vi "Top.vi"(0 "OPC UA client refnum out":T4, 9 "stop":bool, 11 "error IO":errorcluster) -> (3 "Az":T5, 4 "Alt":T6, 6 "HSB":T7, 8 "Fork Panel":T8, 10 "UPS":T10, 15 "Alarm Error":T11)   [LabVIEW 2019]
uses:
  subVIs/Alarm-Ctrl.ctl
  subVIs/UPS-Ctrl.ctl
  <vilib>/OPCUA/controls/NodeId.ctl
  subVIs/Fork Panel-Ctrl.ctl
  subVIs/HSB-Ctrl.ctl
  subVIs/Alt-Ctrl.ctl
  subVIs/Az-Ctrl.ctl
  <vilib>/OPCUA/controls/OPC UA Client Refnum.ctl
  subVIs/Ack-Ctrl.ctl
  <vilib>/OPCUA/controls/Write Variant Request.ctl
  <vilib>/OPCUA/controls/Write Status.ctl
  <vilib>/OPCUA/client/Multiple Write Variant.vi
  <vilib>/OPCUA/NI OPC UA Client.lvlib
panel:
  in  "Alarm_Ack":T1
  in  "UPS_Ack":T2
  in  "FP_Ack":T3
  in  "HSB_Ack":T3
  in  "Alt_Ack":T3
  in  "Az_Ack":T3
  out "node RU":T9[](array[typedef])
  out "node RU 2":T9[](array[typedef])
  out "node RU 3":string[](array[string])
  # "Alarm Error"
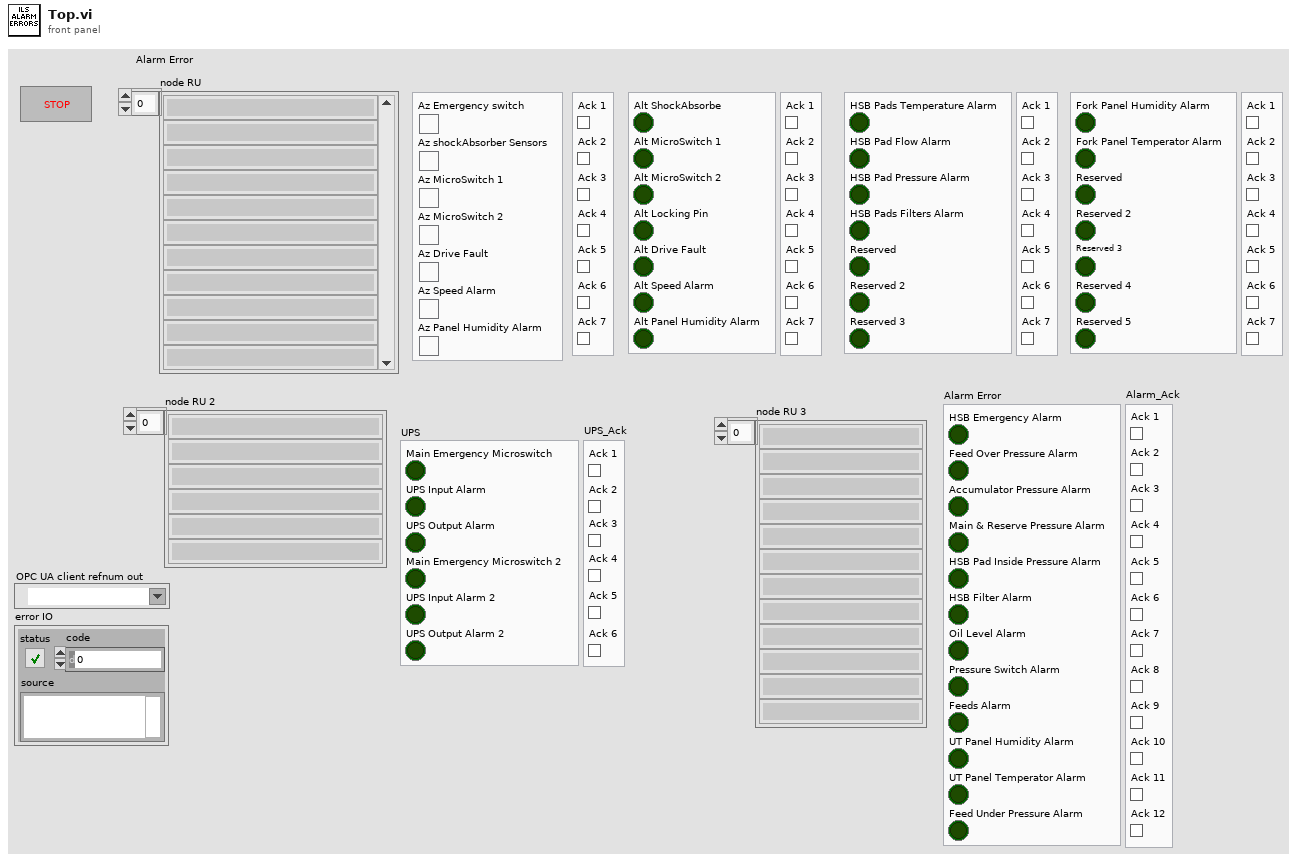
[diagram p1: front panel]
types:
  T1 = cluster{"Ack 1":bool, "Ack 2":bool, "Ack 3":bool, "Ack 4":bool, "Ack 5":bool, "Ack 6":bool, "Ack 7":bool, "Ack 8":bool, "Ack 9":bool, "Ack 10":bool, "Ack 11":bool, "Ack 12":bool}
  T2 = cluster{"Ack 1":bool, "Ack 2":bool, "Ack 3":bool, "Ack 4":bool, "Ack 5":bool, "Ack 6":bool}
  T3 = typedef "Ack-Ctrl.ctl" = cluster{"Ack 1":bool, "Ack 2":bool, "Ack 3":bool, "Ack 4":bool, "Ack 5":bool, "Ack 6":bool, "Ack 7":bool}
  T4 = typedef "OPC UA Client Refnum.ctl" = refnum<k21>
  T5 = typedef "Az-Ctrl.ctl" = cluster{"Az Emergency switch":bool, "Az shockAbsorber Sensors":bool, "Az MicroSwitch 1":bool, "Az MicroSwitch 2":bool, "Az Drive Fault":bool, "Az Speed Alarm":bool, "Az Panel Humidity Alarm":bool}
  T6 = typedef "Alt-Ctrl.ctl" = cluster{"Alt ShockAbsorbe":bool, "Alt MicroSwitch 1":bool, "Alt MicroSwitch 2":bool, "Alt Locking Pin":bool, "Alt Drive Fault":bool, "Alt Speed Alarm":bool, "Alt Panel Humidity Alarm":bool}
  T7 = typedef "HSB-Ctrl.ctl" = cluster{"HSB Pads Temperature Alarm":bool, "HSB Pad Flow Alarm":bool, "HSB Pad Pressure Alarm":bool, "HSB Pads Filters Alarm":bool, "Reserved":bool, "Reserved 2":bool, "Reserved 3":bool}
  T8 = typedef "Fork Panel-Ctrl.ctl" = cluster{"Fork Panel Humidity Alarm":bool, "Fork Panel Temperator Alarm":bool, "Reserved":bool, "Reserved 2":bool, "Reserved 3":bool, "Reserved 4":bool, "Reserved 5":bool}
  T9 = typedef "NodeId.ctl" = string
  T10 = typedef "UPS-Ctrl.ctl" = cluster{"Main Emergency Microswitch":bool, "UPS Input Alarm":bool, "UPS Output Alarm":bool, "Main Emergency Microswitch 2":bool, "UPS Input Alarm 2":bool, "UPS Output Alarm 2":bool}
  T11 = typedef "Alarm-Ctrl.ctl" = cluster{"HSB Emergency Alarm":bool, "Feed Over Pressure Alarm":bool, "Accumulator Pressure Alarm":bool, "Main & Reserve Pressure Alarm":bool, "HSB Pad Inside Pressure Alarm":bool, "HSB Filter Alarm":bool, "Oil Level Alarm":bool, "Pressure Switch Alarm":bool, "Feeds Alarm":bool, "UT Panel Humidity Alarm":bool, "UT Panel Temperator Alarm":bool, "Feed Under Pressure Alarm":bool}
  T12 = typedef "Write Variant Request.ctl" = cluster{"node ID":T9, "value":variant, "timestamp (current time)":timestamp, "node status":T13}
  T13 = typedef "Write Status.ctl" = u32
  T14 = typedef "Subscription ID.ctl" = u32
  T15 = typedef "Subscription Data Change.ctl" = cluster{"node ID":T9, " value":variant, "timestamp":timestamp, "data type":T16, "status code":T17}
  T16 = typedef "Data Type.ctl" = u16
  T17 = typedef "OPC UA StatusCode.ctl" = u32
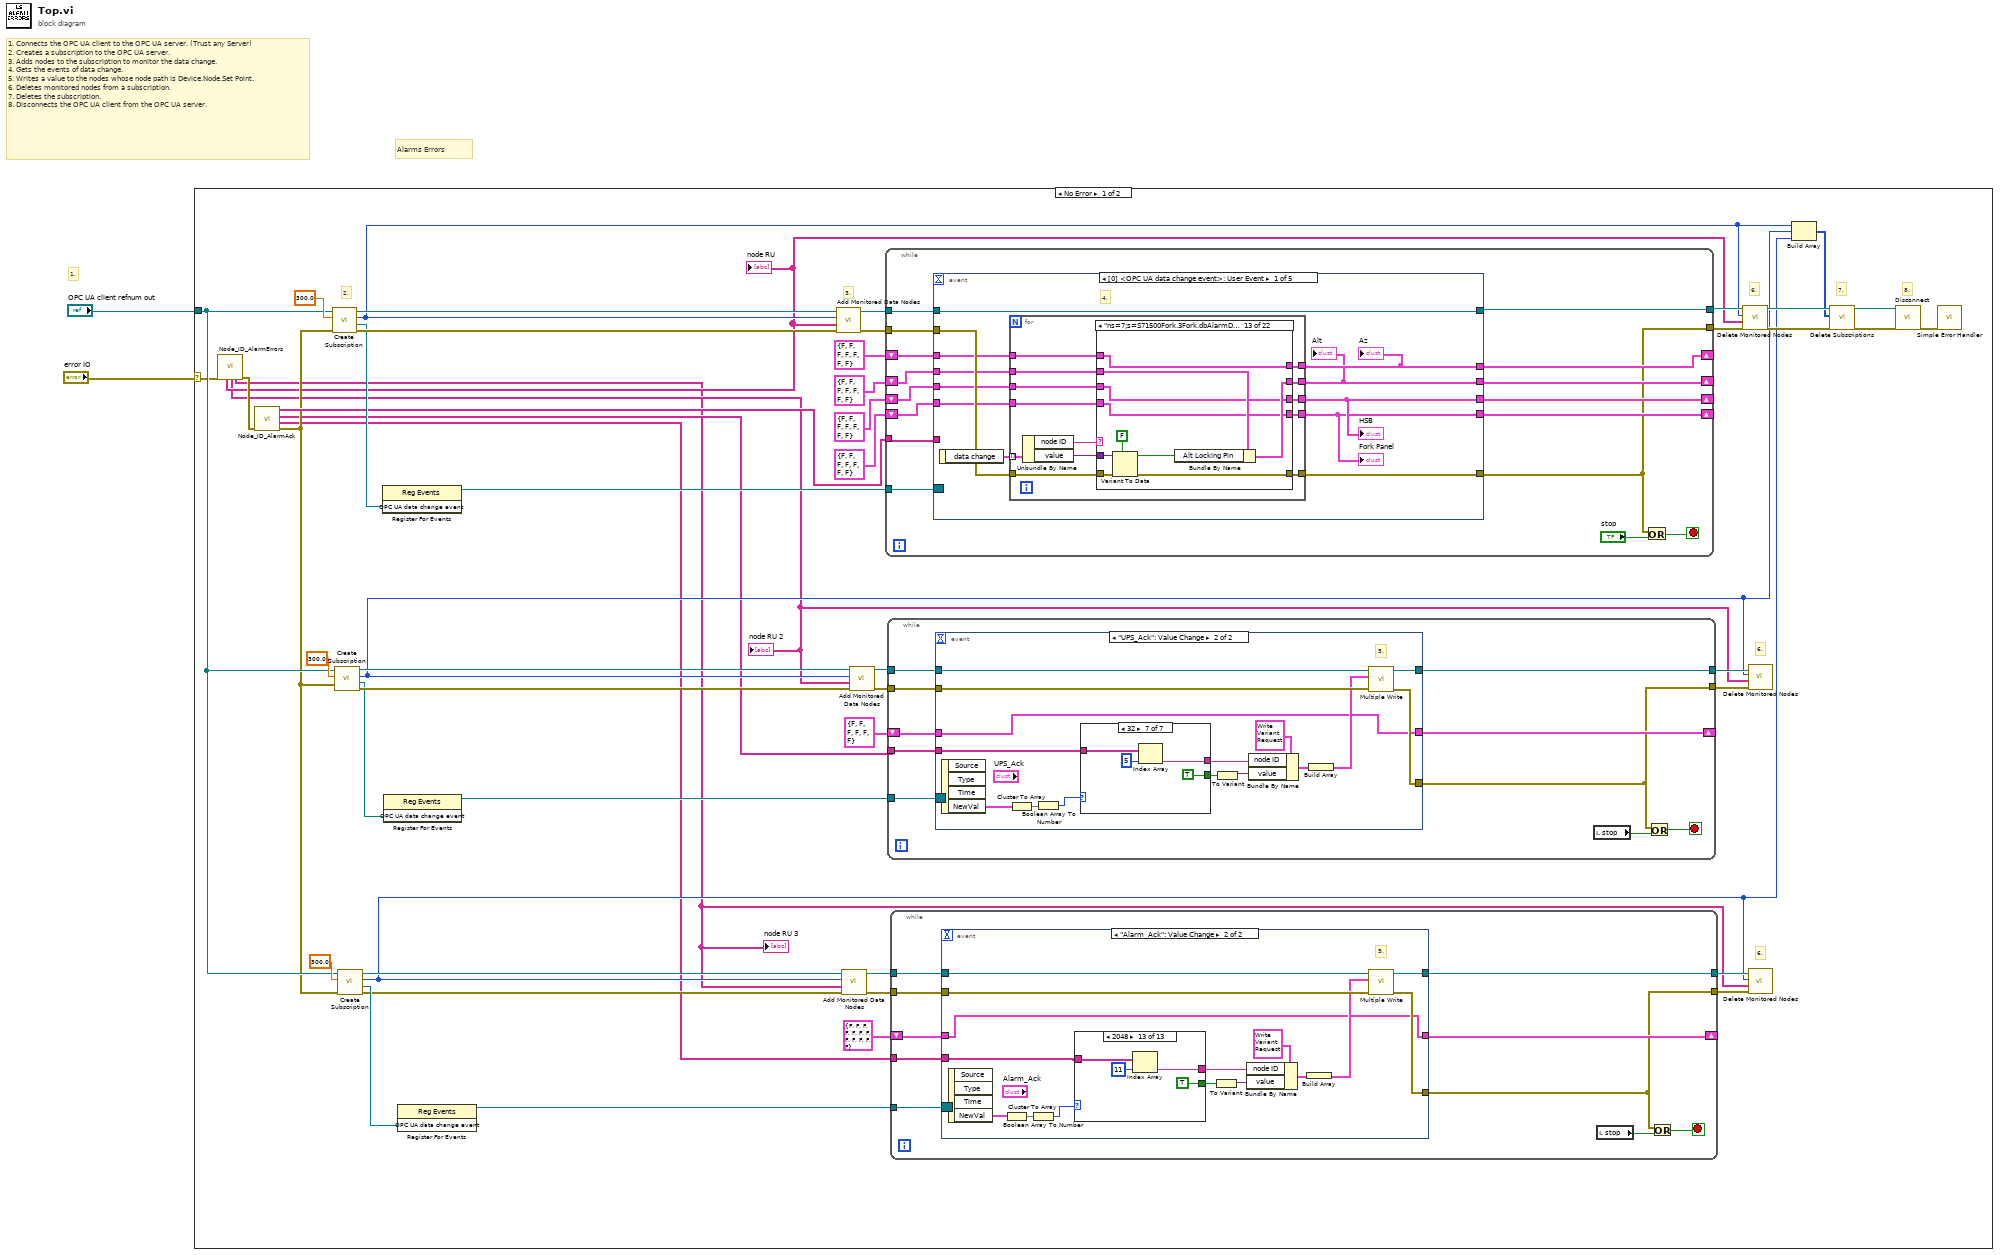
[diagram p0: block diagram]
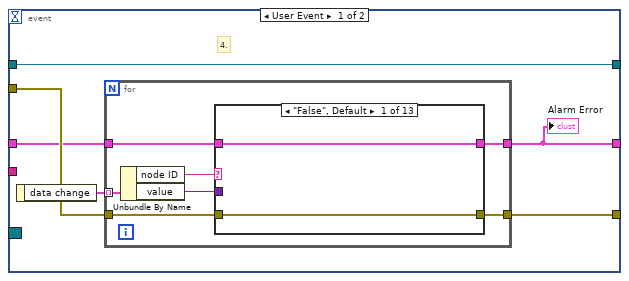
[diagram p2: hidden frame]
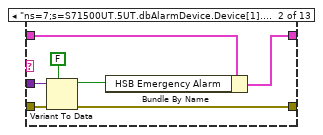
[diagram p3: hidden frame]
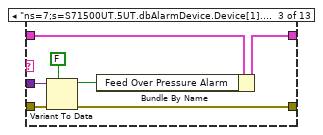
[diagram p4: hidden frame]
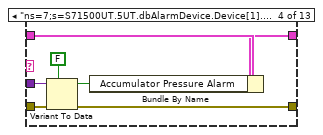
[diagram p5: hidden frame]
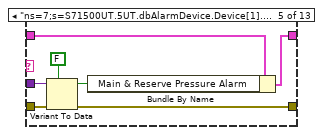
[diagram p6: hidden frame]
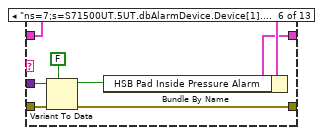
[diagram p7: hidden frame]
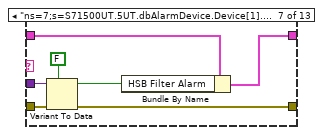
[diagram p8: hidden frame]
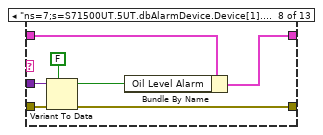
[diagram p9: hidden frame]
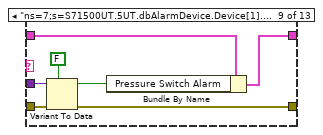
[diagram p10: hidden frame]
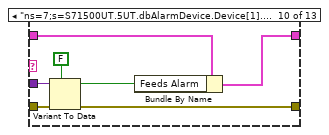
[diagram p11: hidden frame]
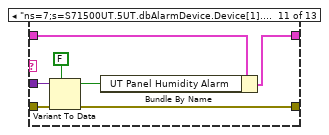
[diagram p12: hidden frame]
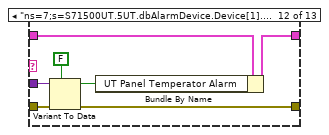
[diagram p13: hidden frame]
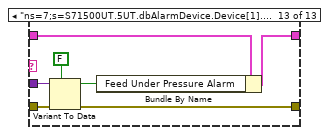
[diagram p14: hidden frame]
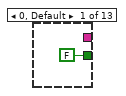
[diagram p15: hidden frame]
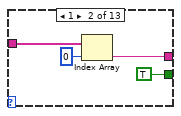
[diagram p16: hidden frame]
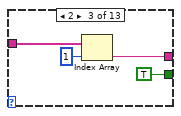
[diagram p17: hidden frame]
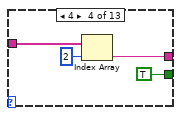
[diagram p18: hidden frame]
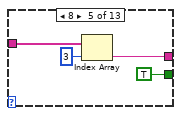
[diagram p19: hidden frame]
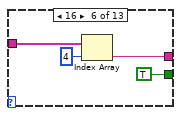
[diagram p20: hidden frame]
diagram:
  # "1."
  # "Alarms Errors"
  # "1. Connects the OPC UA client to the OPC UA server. (Trust any Server) \n2. Creates a subscription to the OPC UA server.\n3. Adds nodes to the subscription to monitor the data change.\n4. Gets the events of data change.\n5. Writes a value to the nodes whose node path is Device.Node.Set Point. \n6. Deletes monitored nodes from a subscription.\n7. Deletes the subscription.\n8. Disconnects the OPC UA client from the OPC UA server."
  n1 = case shown="No Error" "error IO" {
    selector: "error IO" -> [w11 w746]
    tunnel: "OPC UA client refnum out" -> [w24 _]
    frame No Error {
      # "6."
      # "6."
      # "7."
      # "8."
      # "6."
      # "3."
      # "2."
      n2 = call "Node_ID_AlarmErrors.vi"("error in"=w11) -> ("node RU"=w5:T9[], "node RU 2"=w4:T9[], "node RU 3"=w3:string[], "error out"=w9:errorcluster)  [unwired: 8 in, 3 out]
      "node RU" <- w5
      "node RU 2" <- w4
      "node RU 3" <- w3
      n3 = call "Node_ID_AlarmAck.vi"("error in"=w9) -> ("error out"=w8:errorcluster, "node RU 3"=w6:string[], "node RU 2"=w7:T9[], "node RU"=w10:T9[])  [unwired: 7 in]
      n4 = call <vilib>:"Create Subscription.vi"("error in (no error)"=w8, "publishing interval (1000 ms)"=300.0 ("update rate (1000 ms)"), "OPC UA client refnum in"=w24) -> ("error out"=w53:errorcluster, "OPC UA data change event"=w40:refnum<user-event>, "subscription ID out"=w42:T14, "OPC UA client refnum out"=w54:T4)  [unwired: 4 in, 1 out]
      n5 = call <vilib>:"Create Subscription.vi"("error in (no error)"=w8, "publishing interval (1000 ms)"=300.0, "OPC UA client refnum in"=w24) -> ("error out"=w32:errorcluster, "OPC UA data change event"=w30:refnum<user-event>, "subscription ID out"=w26:T14, "OPC UA client refnum out"=w33:T4)  [unwired: 4 in, 1 out]
      n6 = call <vilib>:"Create Subscription.vi"("error in (no error)"=w8, "publishing interval (1000 ms)"=300.0, "OPC UA client refnum in"=w24) -> ("error out"=w21:errorcluster, "OPC UA data change event"=w23:refnum<user-event>, "subscription ID out"=w15:T14, "OPC UA client refnum out"=w22:T4)  [unwired: 4 in, 1 out]
      n7 = register-events(w40) -> (reference out=w52:refnum<event-registration>)  [unwired: 2 in, 1 out]
      n8 = register-events(w30) -> (reference out=w29:refnum<event-registration>)  [unwired: 2 in, 1 out]
      n9 = register-events(w23) -> (reference out=w18:refnum<event-registration>)  [unwired: 2 in, 1 out]
      n10 = call <vilib>:"Add Monitored Data Nodes.vi"("error in (no error)"=w53, "node IDs"=w5, "subscription ID in"=w42, "OPC UA client refnum in"=w54) -> ("error out"=w50:errorcluster, "OPC UA client refnum out"=w51:T4)  [unwired: 4 in, 2 out]
      n11 = call <vilib>:"Add Monitored Data Nodes.vi"("error in (no error)"=w21, "node IDs"=w3, "subscription ID in"=w15, "OPC UA client refnum in"=w22) -> ("error out"=w19:errorcluster, "OPC UA client refnum out"=w20:T4)  [unwired: 4 in, 2 out]
      n12 = call <vilib>:"Add Monitored Data Nodes.vi"("error in (no error)"=w32, "node IDs"=w4, "subscription ID in"=w26, "OPC UA client refnum in"=w33) -> ("error out"=w31:errorcluster, "OPC UA client refnum out"=w14:T4)  [unwired: 4 in, 2 out]
      n13 = while {
        tunnel: w52 -> [w350]
        tunnel: w51 -> [w349]
        tunnel: w50 -> [w348]
        tunnel: [w335] -> w48
        tunnel: [w336] -> w49
        shift-right: [w344] -> _
        shift-left: T5 {"Az Emergency switch"=FALSE, "Az shockAbsorber Sensors"=FALSE, "Az MicroSwitch 1"=FALSE, "Az MicroSwitch 2"=FALSE, "Az Drive Fault"=FALSE, "Az Speed Alarm"=FALSE, "Az Panel Humidity Alarm"=FALSE} ("Az") -> [w345]
        shift-right: [w342] -> _
        shift-left: T6 {"Alt ShockAbsorbe"=FALSE, "Alt MicroSwitch 1"=FALSE, "Alt MicroSwitch 2"=FALSE, "Alt Locking Pin"=FALSE, "Alt Drive Fault"=FALSE, "Alt Speed Alarm"=FALSE, "Alt Panel Humidity Alarm"=FALSE} ("Cluster") -> [w343]
        shift-right: [w339] -> _
        shift-left: T7 {"HSB Pads Temperature Alarm"=FALSE, "HSB Pad Flow Alarm"=FALSE, "HSB Pad Pressure Alarm"=FALSE, "HSB Pads Filters Alarm"=FALSE, "Reserved"=FALSE, "Reserved 2"=FALSE, "Reserved 3"=FALSE} ("HSB") -> [w341]
        shift-right: [w338] -> _
        shift-left: T8 {"Fork Panel Humidity Alarm"=FALSE, "Fork Panel Temperator Alarm"=FALSE, "Reserved"=FALSE, "Reserved 2"=FALSE, "Reserved 3"=FALSE, "Reserved 4"=FALSE, "Reserved 5"=FALSE} ("Fork Panel") -> [w340]
        tunnel: w10 -> [w337]
        stop <- w347 stop-if-true
        n14 = event shown="[0] <OPC UA data change event>: User Event" {
          selector: w350 -> [_ _ _ _ _]
          dyn-events: _ -> [_ _ _ _ _]
          timeout: _ -> [_ _ _ _ _]
          tunnel: w349 -> [w359 w594 w639 w684 w720]
          tunnel: [w359 w595 w640 w685 w721] -> w336
          tunnel: [w360 _ _ _ _] -> w335
          tunnel: w348 -> [w361 _ _ _ _]
          tunnel: w345 -> [w358 w593 w638 w683 w719]
          tunnel: [w357 w593 w638 w683 w719] -> w344
          tunnel: w343 -> [w356 w592 w637 w682 w718]
          tunnel: [w355 w592 w637 w682 w718] -> w342
          tunnel: w341 -> [w354 w591 w636 w681 w717]
          tunnel: w340 -> [w353 w590 w635 w680 w716]
          tunnel: [w352 w591 w636 w681 w717] -> w339
          tunnel: [w351 w590 w635 w680 w716] -> w338
          tunnel: w337 -> [_ w601 w646 w691 w727]
          event User Event {
            # "4."
            n15 = event-data() -> ("data change"=w362:T15[])  [unwired: 1 in]
            n16 = for {
              tunnel: w362 -> [w372] mode=indexing
              tunnel: w361 -> [w374]
              tunnel: [w373] -> w360
              tunnel: w358 -> [w370]
              tunnel: [w369] -> w357
              tunnel: w356 -> [w368]
              tunnel: [w367] -> w355
              tunnel: w354 -> [w366]
              tunnel: w353 -> [w364]
              tunnel: [w365] -> w352
              tunnel: [w363] -> w351
              n17 = Unbundle By Name(w372) -> ("node ID"=w371:T9, "value"=w375:variant)
              n18 = case shown="\"ns=7;s=S71500Fork.3Fork.dbAlarmDevice.Device[2].bAlarmError5\"" w371 {
                tunnel: w375 -> [_ w390 w400 w410 w420 w428 w438 w448 w458 w468 w478 w488 w498 w508 w518 w528 w538 w548 w558 w568 w578 w588]
                tunnel: w374 -> [w380 w388 w398 w408 w418 w426 w436 w446 w456 w466 w476 w486 w496 w506 w516 w526 w536 w546 w556 w566 w576 w586]
                tunnel: [w380 w387 w397 w407 w417 w425 w435 w445 w455 w465 w475 w485 w495 w505 w515 w525 w535 w545 w555 w565 w575 w585] -> w373
                tunnel: w370 -> [w379 w386 w396 w406 w416 w424 w434 w444 w454 w462 w472 w482 w492 w502 w512 w522 w533 w543 w553 w563 w573 w583]
                tunnel: [w379 w385 w395 w405 w415 w424 w433 w443 w453 w462 w472 w482 w492 w502 w512 w522 w533 w543 w553 w563 w573 w583] -> w369
                tunnel: w368 -> [w378 w383 w393 w403 w413 w423 w431 w441 w451 w463 w473 w483 w493 w503 w513 w523 w532 w542 w552 w562 w572 w582]
                tunnel: [w378 w383 w393 w403 w413 w423 w431 w441 w451 w461 w471 w481 w491 w501 w511 w521 w532 w542 w552 w562 w572 w582] -> w367
                tunnel: w366 -> [w377 w382 w392 w402 w412 w422 w430 w440 w450 w460 w470 w480 w490 w500 w510 w520 w531 w541 w551 w561 w571 w581]
                tunnel: [w377 w382 w392 w402 w412 w422 w430 w440 w450 w460 w470 w480 w490 w500 w510 w520 w530 w540 w550 w560 w571 w581] -> w365
                tunnel: w364 -> [w376 w381 w391 w401 w411 w421 w429 w439 w449 w459 w469 w479 w489 w499 w509 w519 w529 w539 w549 w559 w570 w580]
                tunnel: [w376 w381 w391 w401 w411 w421 w429 w439 w449 w459 w469 w479 w489 w499 w509 w519 w529 w539 w549 w559 w569 w579] -> w363
                frame "False", Default {
                }
                frame "ns=7;s=S71500Fork.3Fork.dbAlarmDevice.Device[1].bAlarmError1" {
                  n19 = Variant To Data(error in=w388, type=FALSE, Variant=w390) -> (data=w384:bool, error out=w387:errorcluster)
                  n20 = Bundle By Name(cluster=w386, "Az Emergency switch"=w384) -> (w385:T5)
                }
                frame "ns=7;s=S71500Fork.3Fork.dbAlarmDevice.Device[1].bAlarmError2" {
                  n21 = Variant To Data(error in=w398, type=FALSE, Variant=w400) -> (data=w394:bool, error out=w397:errorcluster)
                  n22 = Bundle By Name(cluster=w396, "Az shockAbsorber Sensors"=w394) -> (w395:T5)
                }
                frame "ns=7;s=S71500Fork.3Fork.dbAlarmDevice.Device[1].bAlarmError3" {
                  n23 = Variant To Data(error in=w408, type=FALSE, Variant=w410) -> (data=w404:bool, error out=w407:errorcluster)
                  n24 = Bundle By Name(cluster=w406, "Az MicroSwitch 1"=w404) -> (w405:T5)
                }
                frame "ns=7;s=S71500Fork.3Fork.dbAlarmDevice.Device[1].bAlarmError4" {
                  n25 = Variant To Data(error in=w418, type=FALSE, Variant=w420) -> (data=w414:bool, error out=w417:errorcluster)
                  n26 = Bundle By Name(cluster=w416, "Az MicroSwitch 2"=w414) -> (w415:T5)
                }
                frame "ns=7;s=S71500Fork.3Fork.dbAlarmDevice.Device[1].bAlarmError5" {
                  n27 = Variant To Data(error in=w426, type=FALSE, Variant=w428) -> (error out=w425:errorcluster)  [unwired: 1 out]
                }
                frame "ns=7;s=S71500Fork.3Fork.dbAlarmDevice.Device[1].bAlarmError6" {
                  n28 = Variant To Data(error in=w436, type=FALSE, Variant=w438) -> (data=w432:bool, error out=w435:errorcluster)
                  n29 = Bundle By Name(cluster=w434, "Az Drive Fault"=w432) -> (w433:T5)
                }
                frame "ns=7;s=S71500Fork.3Fork.dbAlarmDevice.Device[1].bAlarmError7" {
                  n30 = Variant To Data(error in=w446, type=FALSE, Variant=w448) -> (data=w442:bool, error out=w445:errorcluster)
                  n31 = Bundle By Name(cluster=w444, "Az Speed Alarm"=w442) -> (w443:T5)
                }
                frame "ns=7;s=S71500Fork.3Fork.dbAlarmDevice.Device[1].bAlarmError8" {
                  n32 = Variant To Data(error in=w456, type=FALSE, Variant=w458) -> (data=w452:bool, error out=w455:errorcluster)
                  n33 = Bundle By Name(cluster=w454, "Az Panel Humidity Alarm"=w452) -> (w453:T5)
                }
                frame "ns=7;s=S71500Fork.3Fork.dbAlarmDevice.Device[2].bAlarmError2" {
                  n34 = Variant To Data(error in=w466, type=FALSE, Variant=w468) -> (data=w464:bool, error out=w465:errorcluster)
                  n35 = Bundle By Name(cluster=w463, "Alt ShockAbsorbe"=w464) -> (w461:T6)
                }
                frame "ns=7;s=S71500Fork.3Fork.dbAlarmDevice.Device[2].bAlarmError3" {
                  n36 = Variant To Data(error in=w476, type=FALSE, Variant=w478) -> (data=w474:bool, error out=w475:errorcluster)
                  n37 = Bundle By Name(cluster=w473, "Alt MicroSwitch 1"=w474) -> (w471:T6)
                }
                frame "ns=7;s=S71500Fork.3Fork.dbAlarmDevice.Device[2].bAlarmError4" {
                  n38 = Variant To Data(error in=w486, type=FALSE, Variant=w488) -> (data=w484:bool, error out=w485:errorcluster)
                  n39 = Bundle By Name(cluster=w483, "Alt MicroSwitch 2"=w484) -> (w481:T6)
                }
                frame "ns=7;s=S71500Fork.3Fork.dbAlarmDevice.Device[2].bAlarmError5" {
                  n40 = Variant To Data(error in=w496, type=FALSE, Variant=w498) -> (data=w494:bool, error out=w495:errorcluster)
                  n41 = Bundle By Name(cluster=w493, "Alt Locking Pin"=w494) -> (w491:T6)
                }
                frame "ns=7;s=S71500Fork.3Fork.dbAlarmDevice.Device[2].bAlarmError6" {
                  n42 = Variant To Data(error in=w506, type=FALSE, Variant=w508) -> (data=w504:bool, error out=w505:errorcluster)
                  n43 = Bundle By Name(cluster=w503, "Alt Drive Fault"=w504) -> (w501:T6)
                }
                frame "ns=7;s=S71500Fork.3Fork.dbAlarmDevice.Device[2].bAlarmError7" {
                  n44 = Variant To Data(error in=w516, type=FALSE, Variant=w518) -> (data=w514:bool, error out=w515:errorcluster)
                  n45 = Bundle By Name(cluster=w513, "Alt Speed Alarm"=w514) -> (w511:T6)
                }
                frame "ns=7;s=S71500Fork.3Fork.dbAlarmDevice.Device[2].bAlarmError8" {
                  n46 = Variant To Data(error in=w526, type=FALSE, Variant=w528) -> (data=w524:bool, error out=w525:errorcluster)
                  n47 = Bundle By Name(cluster=w523, "Alt Panel Humidity Alarm"=w524) -> (w521:T6)
                }
                frame "ns=7;s=S71500Fork.3Fork.dbAlarmDevice.Device[3].bAlarmError2" {
                  n48 = Variant To Data(error in=w536, type=FALSE, Variant=w538) -> (data=w534:bool, error out=w535:errorcluster)
                  n49 = Bundle By Name(cluster=w531, "HSB Pads Temperature Alarm"=w534) -> (w530:T7)
                }
                frame "ns=7;s=S71500Fork.3Fork.dbAlarmDevice.Device[3].bAlarmError3" {
                  n50 = Variant To Data(error in=w546, type=FALSE, Variant=w548) -> (data=w544:bool, error out=w545:errorcluster)
                  n51 = Bundle By Name(cluster=w541, "HSB Pad Flow Alarm"=w544) -> (w540:T7)
                }
                frame "ns=7;s=S71500Fork.3Fork.dbAlarmDevice.Device[3].bAlarmError4" {
                  n52 = Variant To Data(error in=w556, type=FALSE, Variant=w558) -> (data=w554:bool, error out=w555:errorcluster)
                  n53 = Bundle By Name(cluster=w551, "HSB Pad Pressure Alarm"=w554) -> (w550:T7)
                }
                frame "ns=7;s=S71500Fork.3Fork.dbAlarmDevice.Device[3].bAlarmError5" {
                  n54 = Variant To Data(error in=w566, type=FALSE, Variant=w568) -> (data=w564:bool, error out=w565:errorcluster)
                  n55 = Bundle By Name(cluster=w561, "HSB Pads Filters Alarm"=w564) -> (w560:T7)
                }
                frame "ns=7;s=S71500Fork.3Fork.dbAlarmDevice.Device[4].bAlarmError8" {
                  n56 = Variant To Data(error in=w576, type=FALSE, Variant=w578) -> (data=w574:bool, error out=w575:errorcluster)
                  n57 = Bundle By Name(cluster=w570, "Fork Panel Humidity Alarm"=w574) -> (w569:T8)
                }
                frame "ns=7;s=S71500Fork.3Fork.dbAlarmDevice.Device[4].bAlarmError9" {
                  n58 = Variant To Data(error in=w586, type=FALSE, Variant=w588) -> (data=w584:bool, error out=w585:errorcluster)
                  n59 = Bundle By Name(cluster=w580, "Fork Panel Temperator Alarm"=w584) -> (w579:T8)
                }
              }
            }
            "Az" <- w357
            "Alt" <- w355
            "HSB" <- w352
            "Fork Panel" <- w351
          }
          event Value Change {
            # "5."
            n60 = event-data() -> ("NewVal"=w604:T3)  [unwired: 1 in, 3 out]
            n61 = Cluster To Array(cluster=w604) -> (array=w603:bool[])
            n62 = Boolean Array To Number(Boolean array=w603) -> (number=w602:u32)
            n63 = case shown="64" w602 {
              tunnel: w601 -> [_ w609 w613 w617 w621 w625 w629 w633]
              tunnel: [_ w608 w612 w616 w620 w624 w628 w632] -> w596
              tunnel: [FALSE TRUE TRUE TRUE TRUE TRUE TRUE TRUE] -> w589
              frame 0, Default {
              }
              frame 1 {
                n64 = Index Array(array=w609, index=0) -> (element=w608:T9)
              }
              frame 2 {
                n65 = Index Array(array=w613, index=1) -> (element=w612:T9)
              }
              frame 4 {
                n66 = Index Array(array=w617, index=2) -> (element=w616:T9)
              }
              frame 8 {
                n67 = Index Array(array=w621, index=3) -> (element=w620:T9)
              }
              frame 16 {
                n68 = Index Array(array=w625, index=5) -> (element=w624:T9)
              }
              frame 32 {
                n69 = Index Array(array=w629, index=6) -> (element=w628:T9)
              }
              frame 64 {
                n70 = Index Array(array=w633, index=7) -> (element=w632:T9)
              }
            }
            n71 = To Variant(anything=w589) -> (Variant=w597:variant)
            n72 = Bundle By Name(cluster=T12 {"node ID"="", "value"=variant, "timestamp (current time)"=timestamp(0 s since 1904-01-01), "node status"=0} ("request"), "node ID"=w596, "value"=w597) -> (w600:T12)
            n73 = Build Array(w600) -> (w599:T12[])
            n74 = call-poly <vilib>:"Multiple Write.vi"("requests"=w599, "OPC UA client refnum in"=w594) -> ("OPC UA client refnum out"=w595:T4)  [unwired: 6 in, 3 out]
          }
          event Value Change {
            # "5."
            n75 = event-data() -> ("NewVal"=w649:T3)  [unwired: 1 in, 3 out]
            n76 = Cluster To Array(cluster=w649) -> (array=w648:bool[])
            n77 = Boolean Array To Number(Boolean array=w648) -> (number=w647:u32)
            n78 = case shown="1" w647 {
              tunnel: w646 -> [_ w654 w658 w662 w666 w670 w674 w678]
              tunnel: [_ w653 w657 w661 w665 w669 w673 w677] -> w641
              tunnel: [FALSE TRUE TRUE TRUE TRUE TRUE TRUE TRUE] -> w634
              frame 0, Default {
              }
              frame 1 {
                n79 = Index Array(array=w654, index=10) -> (element=w653:T9)
              }
              frame 2 {
                n80 = Index Array(array=w658, index=11) -> (element=w657:T9)
              }
              frame 4 {
                n81 = Index Array(array=w662, index=12) -> (element=w661:T9)
              }
              frame 8 {
                n82 = Index Array(array=w666, index=13) -> (element=w665:T9)
              }
              frame 16 {
                n83 = Index Array(array=w670, index=14) -> (element=w669:T9)
              }
              frame 32 {
                n84 = Index Array(array=w674, index=15) -> (element=w673:T9)
              }
              frame 64 {
                n85 = Index Array(array=w678, index=16) -> (element=w677:T9)
              }
            }
            n86 = To Variant(anything=w634) -> (Variant=w642:variant)
            n87 = Bundle By Name(cluster=T12 {"node ID"="", "value"=variant, "timestamp (current time)"=timestamp(0 s since 1904-01-01), "node status"=0} ("request"), "node ID"=w641, "value"=w642) -> (w645:T12)
            n88 = Build Array(w645) -> (w644:T12[])
            n89 = call-poly <vilib>:"Multiple Write.vi"("requests"=w644, "OPC UA client refnum in"=w639) -> ("OPC UA client refnum out"=w640:T4)  [unwired: 6 in, 3 out]
          }
          event Value Change {
            # "5."
            n90 = event-data() -> ("NewVal"=w694:T3)  [unwired: 1 in, 3 out]
            n91 = Cluster To Array(cluster=w694) -> (array=w693:bool[])
            n92 = Boolean Array To Number(Boolean array=w693) -> (number=w692:u32)
            n93 = case shown="8" w692 {
              tunnel: w691 -> [_ w699 w703 w707 w711 _ _ _]
              tunnel: [_ w698 w702 w706 w710 _ _ _] -> w686
              tunnel: [FALSE TRUE TRUE TRUE TRUE FALSE FALSE FALSE] -> w679
              frame 0, Default {
              }
              frame 1 {
                n94 = Index Array(array=w699, index=19) -> (element=w698:T9)
              }
              frame 2 {
                n95 = Index Array(array=w703, index=20) -> (element=w702:T9)
              }
              frame 4 {
                n96 = Index Array(array=w707, index=21) -> (element=w706:T9)
              }
              frame 8 {
                n97 = Index Array(array=w711, index=22) -> (element=w710:T9)
              }
              frame 16 {
              }
              frame 32 {
              }
              frame 64 {
              }
            }
            n98 = To Variant(anything=w679) -> (Variant=w687:variant)
            n99 = Bundle By Name(cluster=T12 {"node ID"="", "value"=variant, "timestamp (current time)"=timestamp(0 s since 1904-01-01), "node status"=0} ("request"), "node ID"=w686, "value"=w687) -> (w690:T12)
            n100 = Build Array(w690) -> (w689:T12[])
            n101 = call-poly <vilib>:"Multiple Write.vi"("requests"=w689, "OPC UA client refnum in"=w684) -> ("OPC UA client refnum out"=w685:T4)  [unwired: 6 in, 3 out]
          }
          event Value Change {
            # "5."
            n102 = event-data() -> ("NewVal"=w730:T3)  [unwired: 1 in, 3 out]
            n103 = Cluster To Array(cluster=w730) -> (array=w729:bool[])
            n104 = Boolean Array To Number(Boolean array=w729) -> (number=w728:u32)
            n105 = case shown="2" w728 {
              tunnel: w727 -> [_ w735 w739 _ _ _ _ _]
              tunnel: [_ w734 w738 _ _ _ _ _] -> w722
              tunnel: [FALSE TRUE TRUE FALSE FALSE FALSE FALSE FALSE] -> w715
              frame 0, Default {
              }
              frame 1 {
                n106 = Index Array(array=w735, index=34) -> (element=w734:T9)
              }
              frame 2 {
                n107 = Index Array(array=w739, index=35) -> (element=w738:T9)
              }
              frame 4 {
              }
              frame 8 {
              }
              frame 16 {
              }
              frame 32 {
              }
              frame 64 {
              }
            }
            n108 = To Variant(anything=w715) -> (Variant=w723:variant)
            n109 = Bundle By Name(cluster=T12 {"node ID"="", "value"=variant, "timestamp (current time)"=timestamp(0 s since 1904-01-01), "node status"=0} ("request"), "node ID"=w722, "value"=w723) -> (w726:T12)
            n110 = Build Array(w726) -> (w725:T12[])
            n111 = call-poly <vilib>:"Multiple Write.vi"("requests"=w725, "OPC UA client refnum in"=w720) -> ("OPC UA client refnum out"=w721:T4)  [unwired: 6 in, 3 out]
          }
        }
        n112 = Or(x=w335, y="stop") -> (x .or. y?=w347:bool)
      }
      n113 = while {
        tunnel: w29 -> [w237]
        tunnel: w14 -> [w236]
        tunnel: w31 -> [w235]
        shift-right: [w232] -> _
        shift-left: T10 {"Main Emergency Microswitch"=FALSE, "UPS Input Alarm"=FALSE, "UPS Output Alarm"=FALSE, "Main Emergency Microswitch 2"=FALSE, "UPS Input Alarm 2"=FALSE, "UPS Output Alarm 2"=FALSE} ("UPS") -> [w233]
        tunnel: [w231] -> w28
        tunnel: [w230] -> w27
        tunnel: w7 -> [w228]
        stop <- w234 stop-if-true
        n114 = event shown="[1] \"UPS_Ack\": Value Change" {
          selector: w237 -> [_ _]
          dyn-events: _ -> [_ _]
          timeout: _ -> [_ _]
          tunnel: w236 -> [w240 w299]
          tunnel: [w240 w300] -> w231
          tunnel: [w241 w297] -> w230
          tunnel: w235 -> [w242 w298]
          tunnel: w233 -> [w239 w295]
          tunnel: [w238 w295] -> w232
          tunnel: w228 -> [_ w306]
          event User Event {
            # "4."
            n115 = event-data() -> ("data change"=w243:T15[])  [unwired: 1 in]
            n116 = for {
              tunnel: w243 -> [w247] mode=indexing
              tunnel: w242 -> [w249]
              tunnel: [w248] -> w241
              tunnel: w239 -> [w245]
              tunnel: [w244] -> w238
              n117 = Unbundle By Name(w247) -> ("node ID"=w246:T9, "value"=w250:variant)
              n118 = case shown="\"ns=7;s=S71500Main1.1Main1.dbAlarmDevice.Device[1].bAlarmError1\"" w246 {
                tunnel: w250 -> [_ w259 w266 w273 w280 w287 w294]
                tunnel: w249 -> [w252 w257 w264 w271 w278 w285 w292]
                tunnel: [w252 w256 w263 w270 w277 w284 w291] -> w248
                tunnel: w245 -> [w251 w255 w262 w269 w276 w282 w290]
                tunnel: [w251 w253 w261 w268 w275 w281 w289] -> w244
                frame "False", Default {
                }
                frame "ns=7;s=S71500Main1.1Main1.dbAlarmDevice.Device[1].bAlarmError1" {
                  n119 = Variant To Data(error in=w257, type=FALSE, Variant=w259) -> (data=w254:bool, error out=w256:errorcluster)
                  n120 = Bundle By Name(cluster=w255, "Main Emergency Microswitch"=w254) -> (w253:T10)
                }
                frame "ns=7;s=S71500Main1.1Main1.dbAlarmDevice.Device[1].bAlarmError2" {
                  n121 = Variant To Data(error in=w264, type=FALSE, Variant=w266) -> (data=w260:bool, error out=w263:errorcluster)
                  n122 = Bundle By Name(cluster=w262, "UPS Input Alarm"=w260) -> (w261:T10)
                }
                frame "ns=7;s=S71500Main1.1Main1.dbAlarmDevice.Device[1].bAlarmError3" {
                  n123 = Variant To Data(error in=w271, type=FALSE, Variant=w273) -> (data=w267:bool, error out=w270:errorcluster)
                  n124 = Bundle By Name(cluster=w269, "UPS Output Alarm"=w267) -> (w268:T10)
                }
                frame "ns=7;s=S71500Main2.1Main2.dbAlarmDevice.Device[1].bAlarmError1" {
                  n125 = Variant To Data(error in=w278, type=FALSE, Variant=w280) -> (data=w274:bool, error out=w277:errorcluster)
                  n126 = Bundle By Name(cluster=w276, "Main Emergency Microswitch 2"=w274) -> (w275:T10)
                }
                frame "ns=7;s=S71500Main2.1Main2.dbAlarmDevice.Device[1].bAlarmError2" {
                  n127 = Variant To Data(error in=w285, type=FALSE, Variant=w287) -> (data=w283:bool, error out=w284:errorcluster)
                  n128 = Bundle By Name(cluster=w282, "UPS Input Alarm 2"=w283) -> (w281:T10)
                }
                frame "ns=7;s=S71500Main2.1Main2.dbAlarmDevice.Device[1].bAlarmError3" {
                  n129 = Variant To Data(error in=w292, type=FALSE, Variant=w294) -> (data=w288:bool, error out=w291:errorcluster)
                  n130 = Bundle By Name(cluster=w290, "UPS Output Alarm 2"=w288) -> (w289:T10)
                }
              }
            }
            "UPS" <- w238
          }
          event "UPS_Ack": Value Change {
            # "5."
            n131 = event-data() -> ("NewVal"=w308:T2)  [unwired: 1 in, 3 out]
            n132 = Cluster To Array(cluster=w308) -> (array=w309:bool[])
            n133 = Boolean Array To Number(Boolean array=w309) -> (number=w307:u32)
            n134 = case shown="32" w307 {
              tunnel: w306 -> [_ w314 w318 w322 w326 w330 w334]
              tunnel: [_ w313 w317 w321 w325 w329 w333] -> w302
              tunnel: [FALSE TRUE TRUE TRUE TRUE TRUE TRUE] -> w301
              frame 0, Default {
              }
              frame 1 {
                n135 = Index Array(array=w314, index=0) -> (element=w313:T9)
              }
              frame 2 {
                n136 = Index Array(array=w318, index=1) -> (element=w317:T9)
              }
              frame 4 {
                n137 = Index Array(array=w322, index=2) -> (element=w321:T9)
              }
              frame 8 {
                n138 = Index Array(array=w326, index=3) -> (element=w325:T9)
              }
              frame 16 {
                n139 = Index Array(array=w330, index=4) -> (element=w329:T9)
              }
              frame 32 {
                n140 = Index Array(array=w334, index=5) -> (element=w333:T9)
              }
            }
            n141 = To Variant(anything=w301) -> (Variant=w303:variant)
            n142 = Bundle By Name(cluster=T12 {"node ID"="", "value"=variant, "timestamp (current time)"=timestamp(0 s since 1904-01-01), "node status"=0} ("request"), "node ID"=w302, "value"=w303) -> (w305:T12)
            n143 = Build Array(w305) -> (w296:T12[])
            n144 = call-poly <vilib>:"Multiple Write.vi"("error in (no error)"=w298, "requests"=w296, "OPC UA client refnum in"=w299) -> ("error out"=w297:errorcluster, "OPC UA client refnum out"=w300:T4)  [unwired: 5 in, 2 out]
          }
        }
        n145 = local read "stop"() -> (w229:bool)
        n146 = Or(x=w230, y=w229) -> (x .or. y?=w234:bool)
      }
      n147 = while {
        tunnel: w18 -> [w64]
        tunnel: w20 -> [w63]
        tunnel: w19 -> [w62]
        shift-right: [w59] -> _
        shift-left: T11 {"HSB Emergency Alarm"=FALSE, "Feed Over Pressure Alarm"=FALSE, "Accumulator Pressure Alarm"=FALSE, "Main & Reserve Pressure Alarm"=FALSE, "HSB Pad Inside Pressure Alarm"=FALSE, "HSB Filter Alarm"=FALSE, "Oil Level Alarm"=FALSE, "Pressure Switch Alarm"=FALSE, "Feeds Alarm"=FALSE, "UT Panel Humidity Alarm"=FALSE, "UT Panel Temperator Alarm"=FALSE, "Feed Under Pressure Alarm"=FALSE} ("Alarm Error") -> [w60]
        tunnel: [w58] -> w17
        tunnel: [w57] -> w16
        tunnel: w6 -> [w55]
        stop <- w61 stop-if-true
        n148 = event shown="[1] \"Alarm_Ack\": Value Change" {
          selector: w64 -> [_ _]
          dyn-events: _ -> [_ _]
          timeout: _ -> [_ _]
          tunnel: w63 -> [w67 w168]
          tunnel: [w67 w169] -> w58
          tunnel: [w68 w166] -> w57
          tunnel: w62 -> [w69 w167]
          tunnel: w60 -> [w66 w164]
          tunnel: [w65 w164] -> w59
          tunnel: w55 -> [_ w175]
          event User Event {
            # "4."
            n149 = event-data() -> ("data change"=w70:T15[])  [unwired: 1 in]
            n150 = for {
              tunnel: w70 -> [w74] mode=indexing
              tunnel: w69 -> [w76]
              tunnel: [w75] -> w68
              tunnel: w66 -> [w72]
              tunnel: [w71] -> w65
              n151 = Unbundle By Name(w74) -> ("node ID"=w73:T9, "value"=w77:variant)
              n152 = case shown="\"False\", Default" w73 {
                tunnel: w77 -> [_ w86 w93 w100 w107 w114 w121 w128 w135 w142 w149 w156 w163]
                tunnel: w76 -> [w79 w84 w91 w98 w105 w112 w119 w126 w133 w140 w147 w154 w161]
                tunnel: [w79 w83 w90 w97 w104 w111 w118 w125 w132 w139 w146 w153 w160] -> w75
                tunnel: w72 -> [w78 w82 w89 w96 w103 w109 w117 w124 w131 w138 w145 w152 w159]
                tunnel: [w78 w80 w88 w95 w102 w108 w116 w123 w130 w137 w144 w151 w158] -> w71
                frame "False", Default {
                }
                frame "ns=7;s=S71500UT.5UT.dbAlarmDevice.Device[1].bAlarmError1" {
                  n153 = Variant To Data(error in=w84, type=FALSE, Variant=w86) -> (data=w81:bool, error out=w83:errorcluster)
                  n154 = Bundle By Name(cluster=w82, "HSB Emergency Alarm"=w81) -> (w80:T11)
                }
                frame "ns=7;s=S71500UT.5UT.dbAlarmDevice.Device[1].bAlarmError2" {
                  n155 = Variant To Data(error in=w91, type=FALSE, Variant=w93) -> (data=w87:bool, error out=w90:errorcluster)
                  n156 = Bundle By Name(cluster=w89, "Feed Over Pressure Alarm"=w87) -> (w88:T11)
                }
                frame "ns=7;s=S71500UT.5UT.dbAlarmDevice.Device[1].bAlarmError3" {
                  n157 = Variant To Data(error in=w98, type=FALSE, Variant=w100) -> (data=w94:bool, error out=w97:errorcluster)
                  n158 = Bundle By Name(cluster=w96, "Accumulator Pressure Alarm"=w94) -> (w95:T11)
                }
                frame "ns=7;s=S71500UT.5UT.dbAlarmDevice.Device[1].bAlarmError4" {
                  n159 = Variant To Data(error in=w105, type=FALSE, Variant=w107) -> (data=w101:bool, error out=w104:errorcluster)
                  n160 = Bundle By Name(cluster=w103, "Main & Reserve Pressure Alarm"=w101) -> (w102:T11)
                }
                frame "ns=7;s=S71500UT.5UT.dbAlarmDevice.Device[1].bAlarmError5" {
                  n161 = Variant To Data(error in=w112, type=FALSE, Variant=w114) -> (data=w110:bool, error out=w111:errorcluster)
                  n162 = Bundle By Name(cluster=w109, "HSB Pad Inside Pressure Alarm"=w110) -> (w108:T11)
                }
                frame "ns=7;s=S71500UT.5UT.dbAlarmDevice.Device[1].bAlarmError6" {
                  n163 = Variant To Data(error in=w119, type=FALSE, Variant=w121) -> (data=w115:bool, error out=w118:errorcluster)
                  n164 = Bundle By Name(cluster=w117, "HSB Filter Alarm"=w115) -> (w116:T11)
                }
                frame "ns=7;s=S71500UT.5UT.dbAlarmDevice.Device[1].bAlarmError7" {
                  n165 = Variant To Data(error in=w126, type=FALSE, Variant=w128) -> (data=w122:bool, error out=w125:errorcluster)
                  n166 = Bundle By Name(cluster=w124, "Oil Level Alarm"=w122) -> (w123:T11)
                }
                frame "ns=7;s=S71500UT.5UT.dbAlarmDevice.Device[1].bAlarmError8" {
                  n167 = Variant To Data(error in=w133, type=FALSE, Variant=w135) -> (data=w129:bool, error out=w132:errorcluster)
                  n168 = Bundle By Name(cluster=w131, "Pressure Switch Alarm"=w129) -> (w130:T11)
                }
                frame "ns=7;s=S71500UT.5UT.dbAlarmDevice.Device[1].bAlarmError9" {
                  n169 = Variant To Data(error in=w140, type=FALSE, Variant=w142) -> (data=w136:bool, error out=w139:errorcluster)
                  n170 = Bundle By Name(cluster=w138, "Feeds Alarm"=w136) -> (w137:T11)
                }
                frame "ns=7;s=S71500UT.5UT.dbAlarmDevice.Device[1].bAlarmError10" {
                  n171 = Variant To Data(error in=w147, type=FALSE, Variant=w149) -> (data=w143:bool, error out=w146:errorcluster)
                  n172 = Bundle By Name(cluster=w145, "UT Panel Humidity Alarm"=w143) -> (w144:T11)
                }
                frame "ns=7;s=S71500UT.5UT.dbAlarmDevice.Device[1].bAlarmError11" {
                  n173 = Variant To Data(error in=w154, type=FALSE, Variant=w156) -> (data=w150:bool, error out=w153:errorcluster)
                  n174 = Bundle By Name(cluster=w152, "UT Panel Temperator Alarm"=w150) -> (w151:T11)
                }
                frame "ns=7;s=S71500UT.5UT.dbAlarmDevice.Device[1].bAlarmError12" {
                  n175 = Variant To Data(error in=w161, type=FALSE, Variant=w163) -> (data=w157:bool, error out=w160:errorcluster)
                  n176 = Bundle By Name(cluster=w159, "Feed Under Pressure Alarm"=w157) -> (w158:T11)
                }
              }
            }
            "Alarm Error" <- w65
          }
          event "Alarm_Ack": Value Change {
            # "5."
            n177 = event-data() -> ("NewVal"=w177:T1)  [unwired: 1 in, 3 out]
            n178 = Cluster To Array(cluster=w177) -> (array=w178:bool[])
            n179 = Boolean Array To Number(Boolean array=w178) -> (number=w176:u32)
            n180 = case shown="2048" w176 {
              tunnel: w175 -> [_ w183 w187 w191 w195 w199 w203 w207 w211 w215 w219 w223 w227]
              tunnel: [_ w182 w186 w190 w194 w198 w202 w206 w210 w214 w218 w222 w226] -> w171
              tunnel: [FALSE TRUE TRUE TRUE TRUE TRUE TRUE TRUE TRUE TRUE TRUE TRUE TRUE] -> w170
              frame 0, Default {
              }
              frame 1 {
                n181 = Index Array(array=w183, index=0) -> (element=w182:string)
              }
              frame 2 {
                n182 = Index Array(array=w187, index=1) -> (element=w186:string)
              }
              frame 4 {
                n183 = Index Array(array=w191, index=2) -> (element=w190:string)
              }
              frame 8 {
                n184 = Index Array(array=w195, index=3) -> (element=w194:string)
              }
              frame 16 {
                n185 = Index Array(array=w199, index=4) -> (element=w198:string)
              }
              frame 32 {
                n186 = Index Array(array=w203, index=5) -> (element=w202:string)
              }
              frame 64 {
                n187 = Index Array(array=w207, index=6) -> (element=w206:string)
              }
              frame 128 {
                n188 = Index Array(array=w211, index=7) -> (element=w210:string)
              }
              frame 256 {
                n189 = Index Array(array=w215, index=8) -> (element=w214:string)
              }
              frame 512 {
                n190 = Index Array(array=w219, index=9) -> (element=w218:string)
              }
              frame 1024 {
                n191 = Index Array(array=w223, index=10) -> (element=w222:string)
              }
              frame 2048 {
                n192 = Index Array(array=w227, index=11) -> (element=w226:string)
              }
            }
            n193 = To Variant(anything=w170) -> (Variant=w172:variant)
            n194 = Bundle By Name(cluster=T12 {"node ID"="", "value"=variant, "timestamp (current time)"=timestamp(0 s since 1904-01-01), "node status"=0} ("request"), "node ID"=w171, "value"=w172) -> (w174:T12)
            n195 = Build Array(w174) -> (w165:T12[])
            n196 = call-poly <vilib>:"Multiple Write.vi"("error in (no error)"=w167, "requests"=w165, "OPC UA client refnum in"=w168) -> ("error out"=w166:errorcluster, "OPC UA client refnum out"=w169:T4)  [unwired: 5 in, 2 out]
          }
        }
        n197 = local read "stop"() -> (w56:bool)
        n198 = Or(x=w57, y=w56) -> (x .or. y?=w61:bool)
      }
      n199 = call <vilib>:"Delete Monitored Nodes.vi"("error in (no error)"=w48, "node IDs"=w5, "subscription ID in"=w42, "OPC UA client refnum in"=w49) -> ("error out"=w46:errorcluster, "OPC UA client refnum out"=w47:T4)  [unwired: 3 in, 3 out]
      n200 = call <vilib>:"Delete Monitored Nodes.vi"("error in (no error)"=w27, "node IDs"=w4, "subscription ID in"=w26, "OPC UA client refnum in"=w28) -> ()  [unwired: 3 in, 5 out]
      n201 = call <vilib>:"Delete Monitored Nodes.vi"("error in (no error)"=w16, "node IDs"=w3, "subscription ID in"=w15, "OPC UA client refnum in"=w17) -> ()  [unwired: 3 in, 5 out]
      n202 = Build Array(w42, w26, w15) -> (w41:T14[])
      n203 = call <vilib>:"Delete Subscriptions.vi"("error in (no error)"=w46, "subscription IDs"=w41, "OPC UA client refnum in"=w47) -> ("error out"=w44:errorcluster, "OPC UA client refnum out"=w45:T4)  [unwired: 6 in, 1 out]
      n204 = call <vilib>:"Disconnect.vi"("error in (no error)"=w44, "OPC UA client refnum in"=w45) -> ("error out"=w36:errorcluster)  [unwired: 9 in]
      n205 = call <vilib>:"Simple Error Handler.vi"("error in (no error)"=w36) -> ()  [unwired: 4 in, 5 out]
    }
    frame Error {
      n206 = Unbundle By Name(w746) -> ("code"=w745:i32)
      n207 = case shown="-356612" w745 {
        frame 0, Default {
        }
        frame -356612 {
          n208 = One Button Dialog(message="A communication problem occurred. Ensure that the OPC UA server that you specify in the server endpoint URL is running and the network between the OPC UA server and the OPC UA client is connectable.") -> ()  [unwired: 1 in, 1 out]
        }
      }
    }
  }
